vi "SCB Host.vi"(6 "stop":bool, 7 "Encoder Radius":dbl=2.0, 8 "Encoder Offset":i16=-1021, 9 "Requested Sample":u8, 10 "Random Change":bool, 11 "Start Sample Change":bool) -> (0 "Encoder Radius Readback":dbl=2.0, 1 "Encoder Destination":i32, 2 "Encoder Position":i32, 3 "Current Sample":u8, 4 "Motor status":bool=TRUE, 5 "Change Complete?":bool)   [LabVIEW 2016]
uses:
  SC2 states.ctl
  Interface states.ctl
panel:
  in  "Rotation Timeout":i32=15000
  out "Monitor State":T1=enum."Wait"
  out "error out":errorcluster
  in  "error in (no error)":errorcluster
  out "SC2 State Control":T2=enum."wait"
  out "Raw Encoder":bool[](array[boolean])
  out "Converted Encoder":bool[](array[boolean])
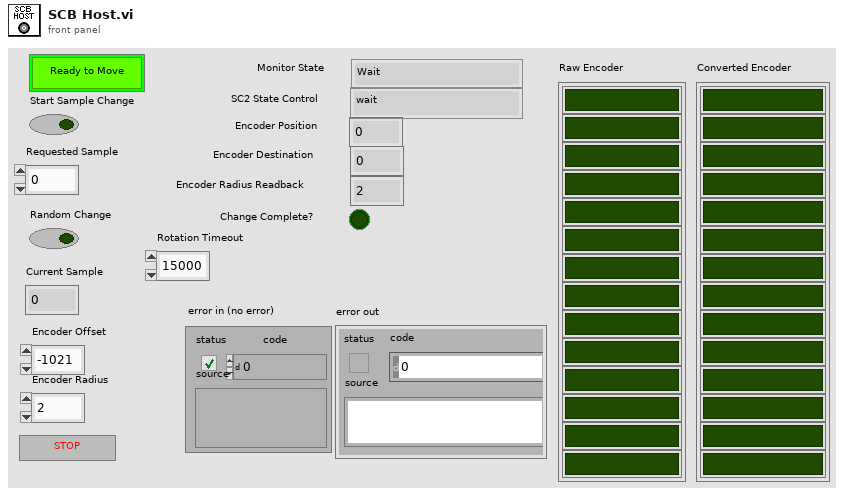
[diagram p1: front panel]
types:
  T1 = typedef "Interface states.ctl" = enum16{"Initialization", "Wait", "start wheel change", "Shutdown"}
  T2 = typedef "SC2 states.ctl" = enum16{"initialize", "wait", "check position", "rotate wheel", "rotate complete", "rotate failure", "Shutdown"}
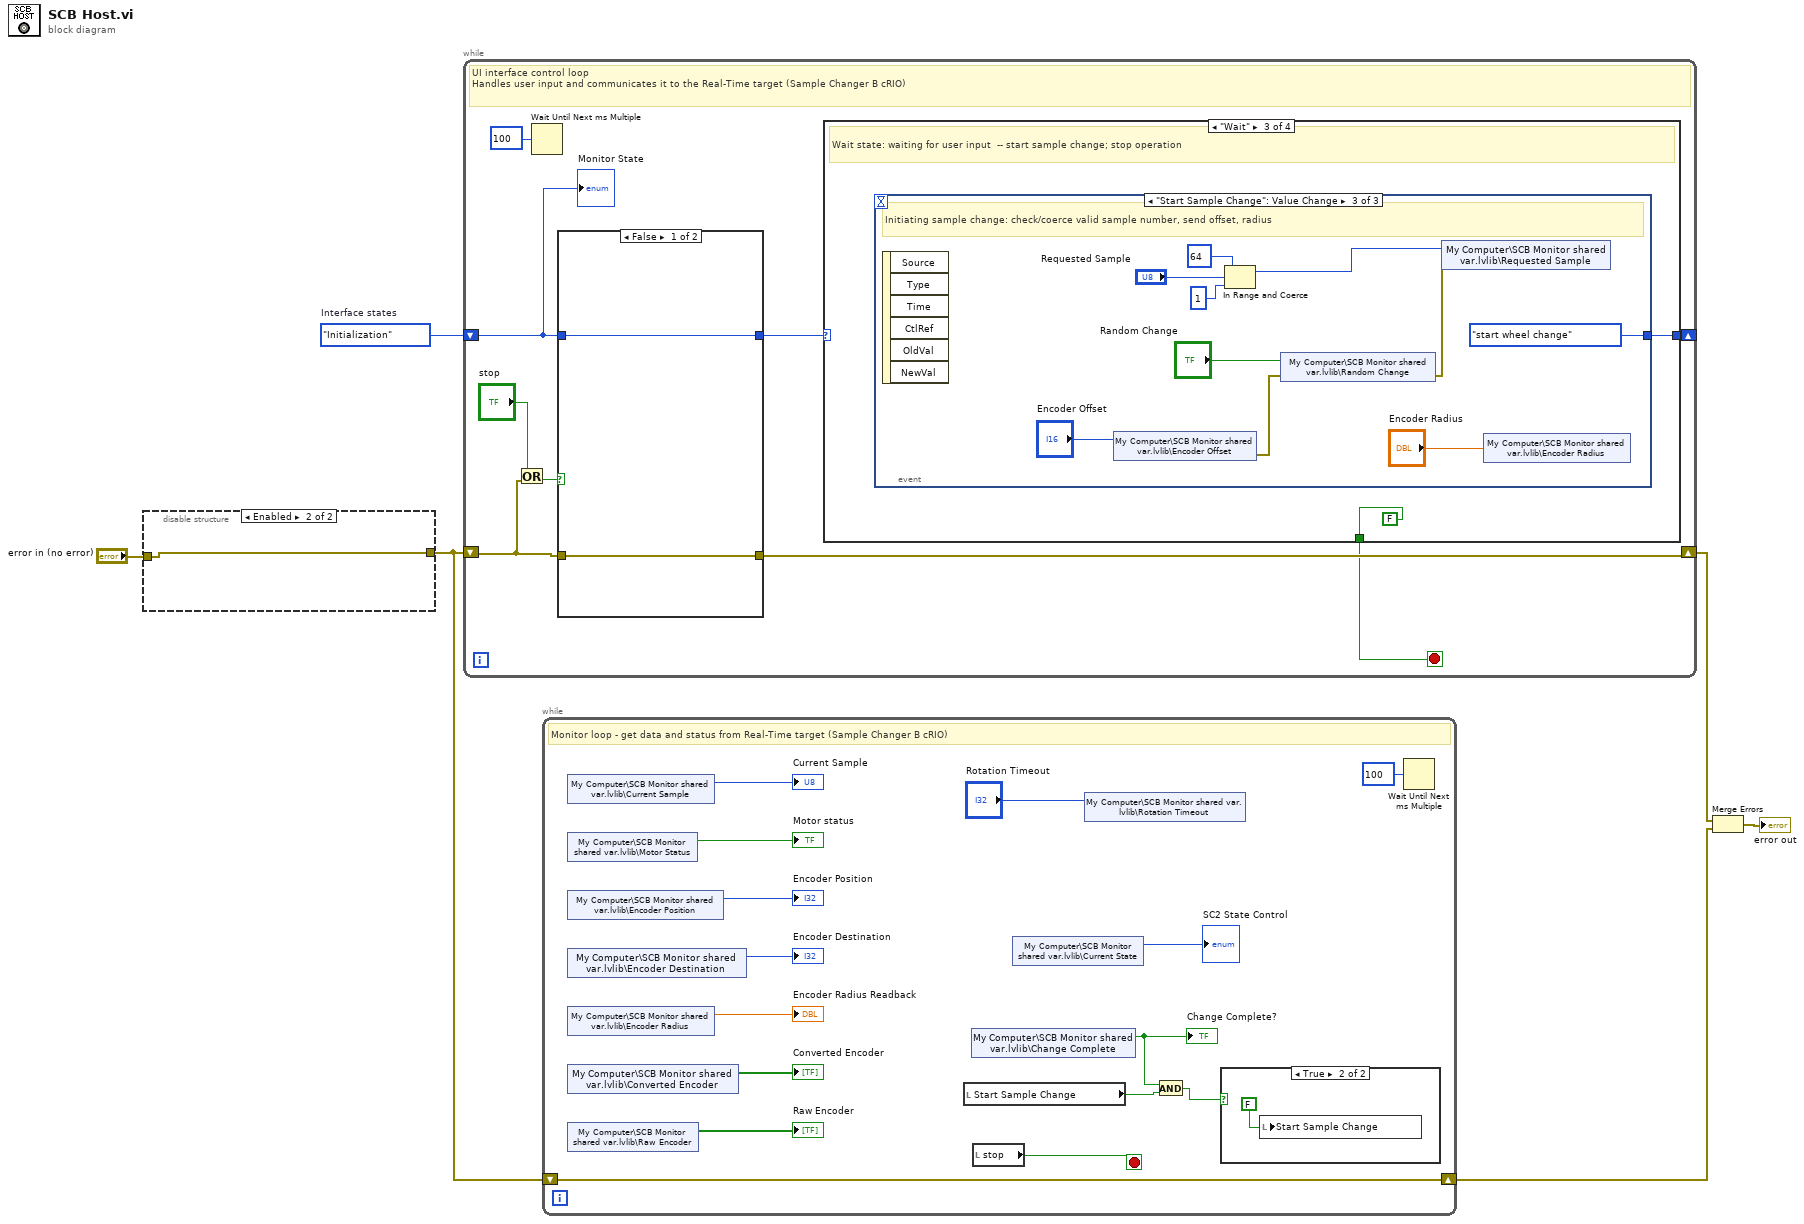
[diagram p0: block diagram]
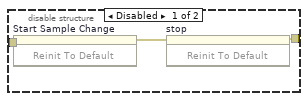
[diagram p2: hidden frame]
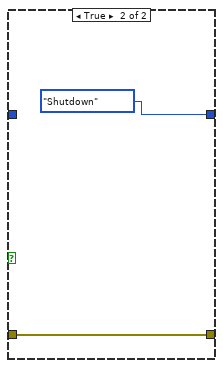
[diagram p4: hidden frame]
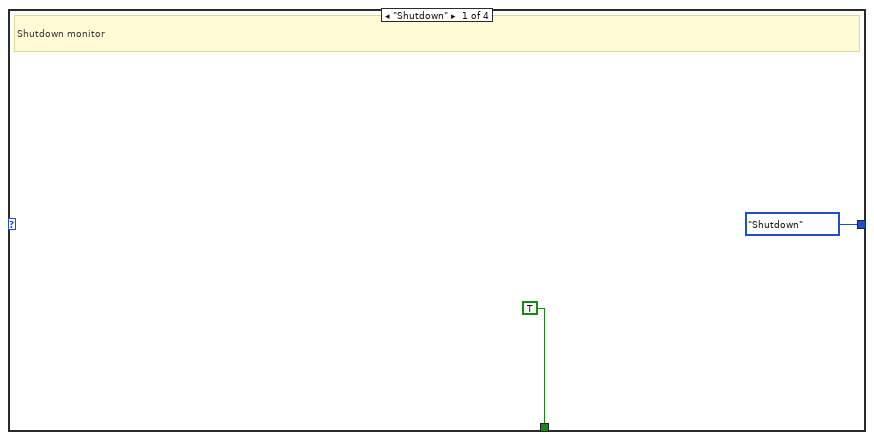
[diagram p5: hidden frame]
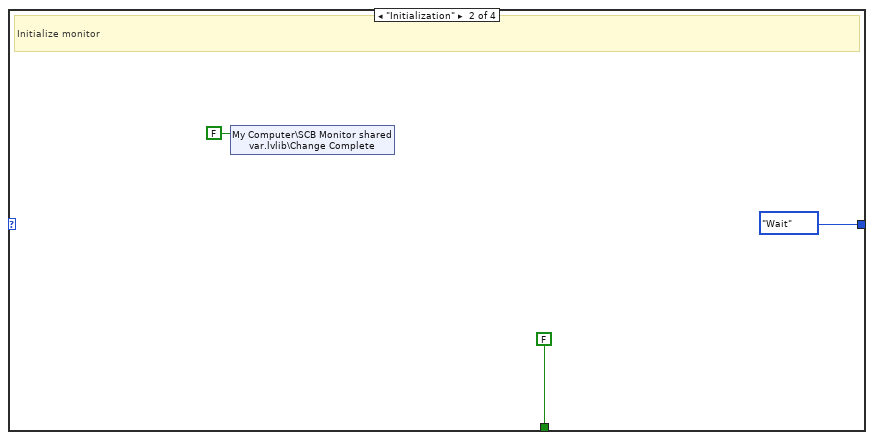
[diagram p6: hidden frame]
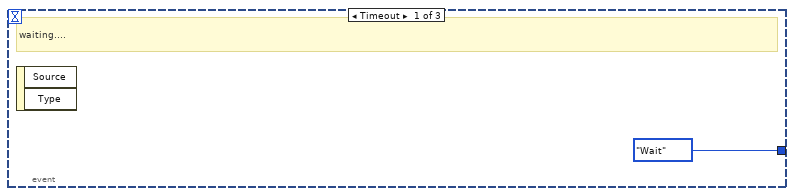
[diagram p7: hidden frame]
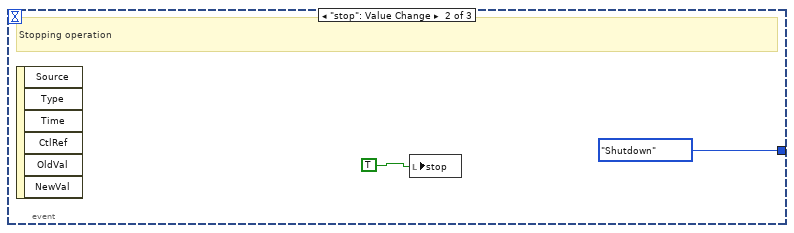
[diagram p8: hidden frame]
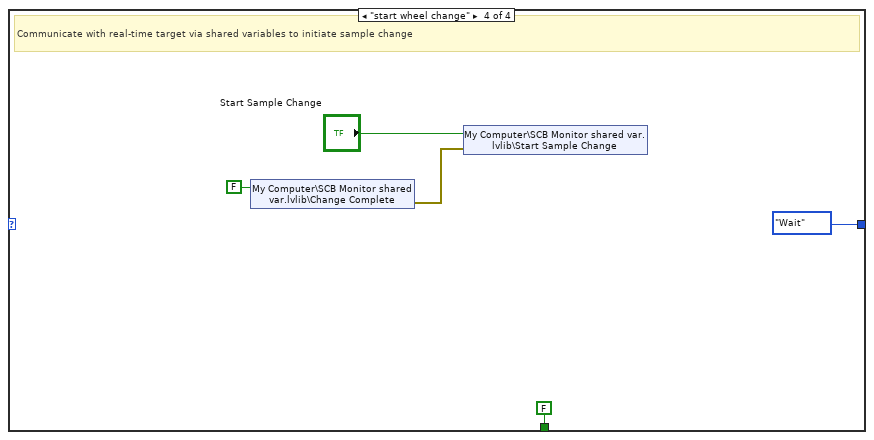
[diagram p9: hidden frame]
diagram:
  w3 = Interface_states."Initialization"  # Interface states
  n1 = disable-structure shown="Enabled" {
    disable-tunnel: [w9 w10] -> w2
    disable-tunnel: "error in (no error)" -> [w7 w10]
    frame Disabled {
      n2 = invoke on="Start Sample Change" class="Bool (strict)" method="Reinit To Default"(error in=w7) -> (error out=w8:errorcluster)  [unwired: 2 in, 2 out]
      n3 = invoke on="stop" class="Bool (strict)" method="Reinit To Default"(error in=w8) -> (error out=w9:errorcluster)  [unwired: 2 in, 2 out]
    }
    frame Enabled {
    }
  }
  n4 = while {
    shift-right: [w16] -> w4
    shift-left: w2 -> [w12]
    shift-right: [w18] -> _
    shift-left: w3 -> [w14]
    stop <- w11 stop-if-true
    # "UI interface control loop\nHandles user input and communicates it to the Real-Time target (Sample Changer B cRIO)"
    n5 = Or(x="stop", y=w12) -> (x .or. y?=w13:bool)
    n6 = Wait Until Next ms Multiple(millisecond multiple=u32 100) -> ()  [unwired: 1 out]
    n7 = case shown="False" w13 {
      tunnel: w12 -> [w21 w22]
      tunnel: [w21 w22] -> w16
      tunnel: [w20 Interface_states."Shutdown" ("Interface states")] -> w15
      tunnel: w14 -> [w20 _]
      frame False {
      }
      frame True {
      }
    }
    n8 = case shown="\"Wait\"" w15 {
      tunnel: [Interface_states."Shutdown" ("Interface states") Interface_states."Wait" ("Interface states") w29 Interface_states."Wait" ("Interface states")] -> w18
      tunnel: [TRUE FALSE FALSE FALSE] -> w11
      frame "Shutdown" {
        # "Shutdown monitor"
      }
      frame "Initialization" {
        # "Initialize monitor"
        n9 = shared-variable "My Computer\\SCB Monitor shared var.lvlib\\Change Complete"(FALSE ("SC2 Change Complete")) -> ()  [unwired: 1 in, 1 out]
      }
      frame "Wait" {
        # "Wait state: waiting for user input  -- start sample change; stop operation"
        n10 = event shown="[2] \"Start Sample Change\": Value Change" {
          selector: _ -> [_ _ _]
          dyn-events: _ -> [_ _ _]
          timeout: _ -> [_ _ _]
          tunnel: [Interface_states."Wait" ("Interface states") Interface_states."Shutdown" ("Interface states") Interface_states."start wheel change" ("Interface states")] -> w29
          event Timeout {
            # "waiting...."
            n11 = event-data() -> ()  [unwired: 1 in, 2 out]
          }
          event "stop": Value Change {
            # "Stopping operation"
            n12 = event-data() -> ()  [unwired: 1 in, 6 out]
            n13 = local write "stop"(TRUE ("stop")) -> ()
          }
          event "Start Sample Change": Value Change {
            # "Initiating sample change: check/coerce valid sample number, send offset, radius"
            n14 = event-data() -> ()  [unwired: 1 in, 6 out]
            n15 = shared-variable "My Computer\\SCB Monitor shared var.lvlib\\Encoder Offset"("Encoder Offset") -> (error out=w35:errorcluster)  [unwired: 1 in]
            n16 = In Range and Coerce(upper limit=u8 64, x="Requested Sample", lower limit=u8 1) -> (coerced(x)=w41:u8)  [unwired: 1 out]
            n17 = shared-variable "My Computer\\SCB Monitor shared var.lvlib\\Random Change"("Random Change", error in=w35) -> (error out=w37:errorcluster)
            n18 = shared-variable "My Computer\\SCB Monitor shared var.lvlib\\Requested Sample"(w41, error in=w37) -> ()  [unwired: 1 out]
            n19 = shared-variable "My Computer\\SCB Monitor shared var.lvlib\\Encoder Radius"("Encoder Radius") -> ()  [unwired: 1 in, 1 out]
          }
        }
      }
      frame "start wheel change" {
        # "Communicate with real-time target via shared variables to initiate sample change"
        n20 = shared-variable "My Computer\\SCB Monitor shared var.lvlib\\Change Complete"(FALSE ("SC2 Change Complete")) -> (error out=w44:errorcluster)  [unwired: 1 in]
        n21 = shared-variable "My Computer\\SCB Monitor shared var.lvlib\\Start Sample Change"("Start Sample Change", error in=w44) -> ()  [unwired: 1 out]
      }
    }
    "Monitor State" <- w14
  }
  n22 = while {
    shift-right: [w62] -> w5
    shift-left: w2 -> [w62]
    stop <- w61 stop-if-true
    # "Monitor loop - get data and status from Real-Time target (Sample Changer B cRIO)"
    n23 = shared-variable "My Computer\\SCB Monitor shared var.lvlib\\Current Sample"() -> (→"Current Sample":u8)  [unwired: 1 in, 1 out]
    n24 = shared-variable "My Computer\\SCB Monitor shared var.lvlib\\Motor Status"() -> (→"Motor status":bool)  [unwired: 1 in, 1 out]
    n25 = shared-variable "My Computer\\SCB Monitor shared var.lvlib\\Encoder Position"() -> (→"Encoder Position":i32)  [unwired: 1 in, 1 out]
    n26 = shared-variable "My Computer\\SCB Monitor shared var.lvlib\\Encoder Destination"() -> (→"Encoder Destination":i32)  [unwired: 1 in, 1 out]
    n27 = shared-variable "My Computer\\SCB Monitor shared var.lvlib\\Encoder Radius"() -> (→"Encoder Radius Readback":dbl)  [unwired: 1 in, 1 out]
    n28 = shared-variable "My Computer\\SCB Monitor shared var.lvlib\\Converted Encoder"() -> (→"Converted Encoder":bool[])  [unwired: 1 in, 1 out]
    n29 = shared-variable "My Computer\\SCB Monitor shared var.lvlib\\Raw Encoder"() -> (→"Raw Encoder":bool[])  [unwired: 1 in, 1 out]
    n30 = local read "Start Sample Change"() -> (w59:bool)
    n31 = shared-variable "My Computer\\SCB Monitor shared var.lvlib\\Change Complete"() -> (w55:bool)  [unwired: 1 in, 1 out]
    "Change Complete?" <- w55
    n32 = local read "stop"() -> (w61:bool)
    n33 = shared-variable "My Computer\\SCB Monitor shared var.lvlib\\Current State"() -> (→"SC2 State Control":u16)  [unwired: 1 in, 1 out]
    n34 = shared-variable "My Computer\\SCB Monitor shared var.lvlib\\Rotation Timeout"("Rotation Timeout") -> ()  [unwired: 1 in, 1 out]
    n35 = And(x=w55, y=w59) -> (x .and. y?=w60:bool)
    n36 = case shown="True" w60 {
      frame False {
      }
      frame True {
        n37 = local write "Start Sample Change"(FALSE ("Start Sample Change")) -> ()
      }
    }
    n38 = Wait Until Next ms Multiple(millisecond multiple=u32 100) -> ()  [unwired: 1 out]
  }
  n39 = Merge Errors(w4, w5) -> (→"error out":errorcluster)
